vi "Open.vi"(8 "error in (no error)":errorcluster, 11 "PythonWrapper in":refnum<class "PythonWrapper.lvclass">) -> (0 "error out":errorcluster, 3 "PythonWrapper out":refnum<class "PythonWrapper.lvclass">)   [LabVIEW 2022 SP3, in "PythonWrapper.lvlib" / "PythonWrapper.lvclass"]
uses:
  PythonWrapper.lvclass
  PythonWrapper.lvclass/PythonWrapper.ctl
  PythonSession/PythonSession.lvclass
  PathUtils/Source/PathUtils.lvlib
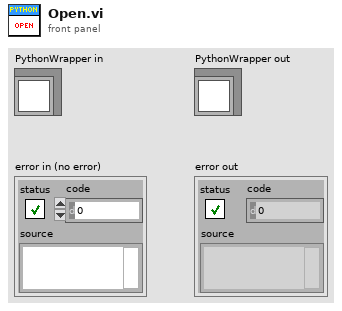
[diagram p1: front panel]
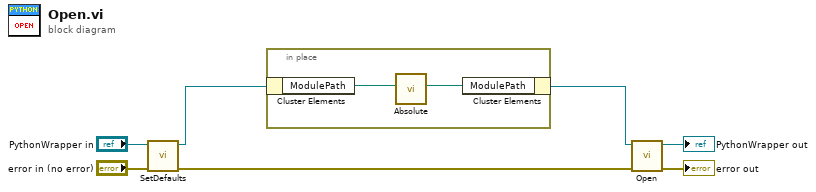
[diagram p0: block diagram]
diagram:
  n1 = call-dynamic "SetDefaults.vi"("error in (no error)"="error in (no error)", "PythonWrapper in"="PythonWrapper in") -> ("error out"=w4:errorcluster, "PythonWrapper out"=w1:refnum<class "PythonWrapper.lvclass">)  [unwired: 8 in]
  n2 = in-place {
    n3 = in-place-cluster #1(w1) -> ("ModulePath"=w9:path)
    n4 = call "Absolute.vi"("Path in"=w9) -> ("Path out"=w8:path)  [unwired: 10 in]
    n5 = in-place-cluster #1("ModulePath"=w8) -> (w2:refnum<class "PythonWrapper.lvclass">)
  }
  n6 = call-parent "Open.vi"("error in (no error)"=w4, "PythonSession in"=w2) -> ("error out"=→"error out":errorcluster, "PythonSession out"=→"PythonWrapper out":refnum<class "PythonWrapper.lvclass">)  [unwired: 8 in]
